vi "Draw Rect Linear Gradient - 3 layers.vi"(9 "Rect":cluster{"horizontal":i16, "vertical":i16}={"horizontal"=400, "vertical"=300}, 10 "Mid Position (%)":i16=70, 11 "Cluster":T1={"Top Color"=16645629, "Mid Color"=14077951, "Bottom Color"=16645629}) -> (3 "2D Picture":picture)   [LabVIEW 2015]
panel:
  out "Benchmark Time (ms)":u32
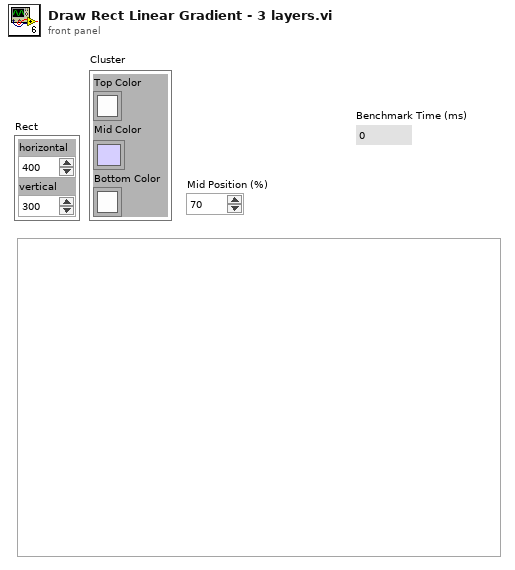
[diagram p1: front panel]
types:
  T1 = cluster{"Top Color":u32, "Mid Color":u32, "Bottom Color":u32}
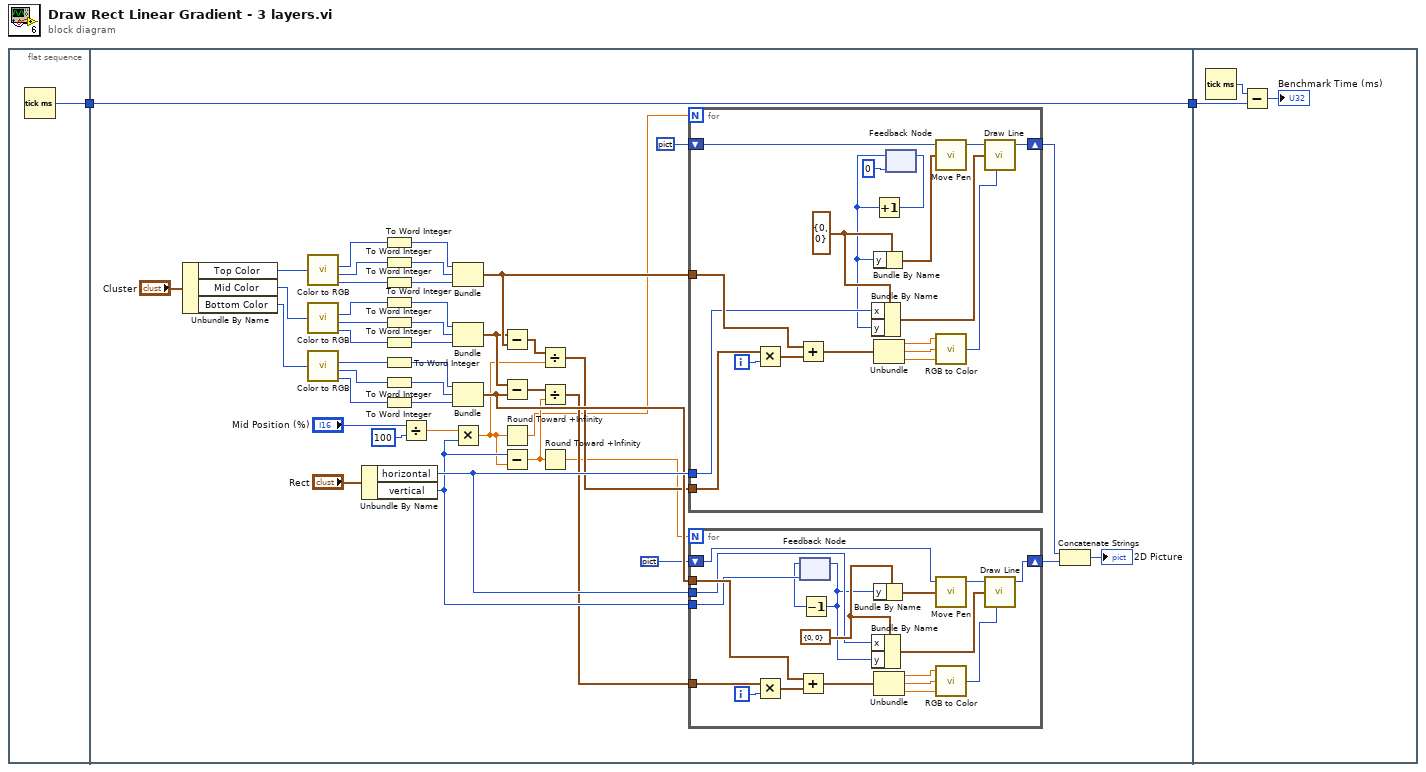
[diagram p0: block diagram]
diagram:
  n1 = flat-sequence {
    tunnel: [w3] -> w1
    tunnel: [w4] -> w2
    tunnel: w1 -> [w4]
    tunnel: w2 -> [w88]
    frame #0 {
      n2 = Tick Count (ms)() -> (millisecond timer value=w3:u32)
    }
    frame #1 {
      n3 = Unbundle By Name("Cluster") -> ("Top Color"=w14:u32, "Mid Color"=w28:u32, "Bottom Color"=w29:u32)
      n4 = call <vilib>:"Color to RGB.vi"("Color"=w14) -> ("R"=w5:u8, "G"=w7:u8, "B"=w8:u8)  [unwired: 1 out]
      n5 = call <vilib>:"Color to RGB.vi"("Color"=w28) -> ("R"=w21:u8, "G"=w20:u8, "B"=w26:u8)  [unwired: 1 out]
      n6 = call <vilib>:"Color to RGB.vi"("Color"=w29) -> ("R"=w22:u8, "G"=w23:u8, "B"=w30:u8)  [unwired: 1 out]
      n7 = Unbundle By Name("Rect") -> ("horizontal"=w48:i16, "vertical"=w47:i16)
      n8 = To Word Integer(number=w5) -> (16bit integer=w17:i16)
      n9 = To Word Integer(number=w7) -> (16bit integer=w16:i16)
      n10 = To Word Integer(number=w8) -> (16bit integer=w15:i16)
      n11 = To Word Integer(number=w21) -> (16bit integer=w18:i16)
      n12 = To Word Integer(number=w20) -> (16bit integer=w19:i16)
      n13 = To Word Integer(number=w26) -> (16bit integer=w27:i16)
      n14 = To Word Integer(number=w22) -> (16bit integer=w25:i16)
      n15 = To Word Integer(number=w23) -> (16bit integer=w24:i16)
      n16 = To Word Integer(number=w30) -> (16bit integer=w31:i16)
      n17 = Divide(x="Mid Position (%)", y=i16 100) -> (x/y=w12:dbl)
      n18 = Bundle(w17, w16, w15) -> (w41:cluster{i16, i16, i16})  [unwired: 1 in]
      n19 = Bundle(w18, w19, w27) -> (w38:cluster{i16, i16, i16})  [unwired: 1 in]
      n20 = Bundle(w25, w24, w31) -> (w46:cluster{i16, i16, i16})  [unwired: 1 in]
      n21 = Multiply(x=w12, y=w47) -> (x*y=w34:dbl)
      n22 = Subtract(x=w38, y=w41) -> (x-y=w6:cluster{i16, i16, i16})
      n23 = Subtract(x=w38, y=w46) -> (x-y=w32:cluster{i16, i16, i16})
      n24 = Round Toward +Infinity(x=w34) -> (ceil(x): smallest int >= x=w35:dbl)
      n25 = Subtract(x=w47, y=w34) -> (x-y=w36:dbl)
      n26 = Divide(x=w6, y=w34) -> (x/y=w40:cluster{dbl, dbl, dbl})
      n27 = Divide(x=w32, y=w36) -> (x/y=w45:cluster{dbl, dbl, dbl})
      n28 = Round Toward +Infinity(x=w36) -> (ceil(x): smallest int >= x=w37:dbl)
      n29 = for {
        N: w35 -> [_]
        shift-right: [w86] -> w42
        shift-left: picture data[5B] ("new picture") -> [w84]
        tunnel: w40 -> [w82]
        tunnel: w41 -> [w80]
        tunnel: w48 -> [w69]
        i -> [w83]
        w71 = cluster{"x":i16, "y":i16} {"x"=0, "y"=0} ("new position")
        n30 = Multiply(x=w82, y=w83) -> (x*y=w81:cluster{dbl, dbl, dbl})
        n31 = Add(x=w80, y=w81) -> (x+y=w79:cluster{dbl, dbl, dbl})
        n32 = Unbundle(w79) -> (w76:dbl, w77:dbl, w78:dbl)
        n33 = feedback #1(i16 0 ("x")) -> (w68:i16)
        n34 = Bundle By Name(cluster=w71, "x"=w69, "y"=w68) -> (w70:cluster{"x":i16, "y":i16})
        n35 = Increment(x=w68) -> (x+1=w73:i16)
        n36 = Bundle By Name(cluster=w71, "y"=w68) -> (w72:cluster{"x":i16, "y":i16})
        n37 = feedback-in #1(w73) -> ()
        n38 = call <vilib>:"Move Pen.vi"("new position"=w72, "picture"=w84) -> ("new picture"=w85:picture)  [unwired: 3 in]
        n39 = call <vilib>:"RGB to Color.vi"("B"=w78, "G"=w77, "R"=w76) -> ("Color"=w75:u32)
        n40 = call <vilib>:"Draw Line.vi"("picture"=w85, "end point"=w70, "color(black)"=w75) -> ("new picture"=w86:picture)  [unwired: 6 in]
      }
      n41 = for {
        N: w37 -> [_]
        shift-right: [w67] -> w43
        shift-left: picture data[5B] ("new picture") -> [w65]
        tunnel: w45 -> [w58]
        tunnel: w46 -> [w57]
        tunnel: w47 -> [w56]
        tunnel: w48 -> [w54]
        i -> [w59]
        w64 = cluster{"x":i16, "y":i16} {"x"=0, "y"=0} ("new position")
        n42 = Multiply(x=w58, y=w59) -> (x*y=w60:cluster{dbl, dbl, dbl})
        n43 = Add(x=w57, y=w60) -> (x+y=w61:cluster{dbl, dbl, dbl})
        n44 = feedback #2(w56) -> (w53:i16)
        n45 = Decrement(x=w53) -> (x-1=w49:i16)
        n46 = feedback-in #2(w49) -> ()
        n47 = Bundle By Name(cluster=w64, "x"=w54, "y"=w49) -> (w52:cluster{"x":i16, "y":i16})
        n48 = Bundle By Name(cluster=w64, "y"=w49) -> (w55:cluster{"x":i16, "y":i16})
        n49 = Unbundle(w61) -> (w63:dbl, w62:dbl, w50:dbl)
        n50 = call <vilib>:"Move Pen.vi"("new position"=w55, "picture"=w65) -> ("new picture"=w66:picture)  [unwired: 3 in]
        n51 = call <vilib>:"RGB to Color.vi"("B"=w50, "G"=w62, "R"=w63) -> ("Color"=w51:u32)
        n52 = call <vilib>:"Draw Line.vi"("picture"=w66, "end point"=w52, "color(black)"=w51) -> ("new picture"=w67:picture)  [unwired: 6 in]
      }
      n53 = Concatenate Strings(w42, w43) -> (→"2D Picture":picture)
    }
    frame #2 {
      n54 = Tick Count (ms)() -> (millisecond timer value=w87:u32)
      n55 = Subtract(x=w87, y=w88) -> (x-y=→"Benchmark Time (ms)":u32)
    }
  }
